vi "AWS_String to TimeStamp.vi"(10 "Input String Array":string[](array[string])) -> (2 "Timestamp":timestamp[](array[timestamp]))   [LabVIEW 2014]
panel:
  out "concatenated string":string
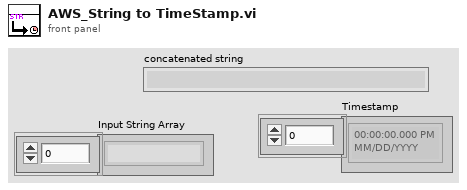
[diagram p1: front panel]
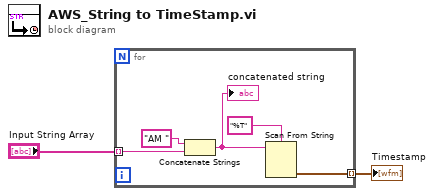
[diagram p0: block diagram]
diagram:
  n1 = for {
    tunnel: "Input String Array" -> [w4] mode=indexing
    tunnel: [w3] -> w1 mode=indexing
    n2 = Concatenate Strings("AM " ("string"), w4) -> (w7:string)
    "concatenated string" <- w7
    n3 = Scan From String(format string="%T", input string=w7) -> (output 1=w3:timestamp)  [unwired: 3 in, 3 out]
  }
  "Timestamp" <- w1
